vi "IsTimeToLaunchGSW__slk_mt.vi"(8 "error in (no error)":errorcluster) -> (0 "error out":errorcluster, 3 "ready?":bool)   [LabVIEW 2020]
doc: "Checks if it is ready to launch GSW."
panel:
  # "IsTimeToLaunchGSW__slk_mt.vi\nChecks if it is ready to launch GSW.\n\nNOTICE -- YOU MUST LEAVE THIS NOTICE IN PLACE.\n\nCopyright (c) 2011, LIANG LIU Shawn.Liu.cn@gmail.com\nAll rights reserved.\n\nRedistribution and use in source and binary forms, with or without modification, are permitted provided that the following conditions are met:\n-Redistributions of source code must retain the above copyright notice, this list of conditions and the following disclaimer.\n-Redistributions in binary form must reproduce the above copyright notice, this list of conditions and the following disclaimer in the documentation and/or other materials provided with the distribution.\n-Neither the name of the eLp nor the names of its contributors may be used to endorse or promote products derived from this software without specific prior written permission.\n\nTHIS SOFTWARE IS PROVIDED BY THE COPYRIGHT HOLDERS AND CONTRIBUTORS \"AS IS\" AND ANY EXPRESS OR IMPLIED WARRANTIES, INCLUDING, BUT NOT LIMITED TO, THE IMPLIED WARRANTIES OF MERCHANTABILITY AND FITNESS FOR A PARTICULAR PURPOSE ARE DISCLAIMED. IN NO EVENT SHALL THE COPYRIGHT HOLDER OR CONTRIBUTORS BE LIABLE FOR ANY DIRECT, INDIRECT, INCIDENTAL, SPECIAL, EXEMPLARY, OR CONSEQUENTIAL DAMAGES (INCLUDING, BUT NOT LIMITED TO, PROCUREMENT OF SUBSTITUTE GOODS OR SERVICES; LOSS OF USE, DATA, OR PROFITS; OR BUSINESS INTERRUPTION) HOWEVER CAUSED AND ON ANY THEORY OF LIABILITY, WHETHER IN CONTRACT, STRICT LIABILITY, OR TORT (INCLUDING NEGLIGENCE OR OTHERWISE) ARISING IN ANY WAY OUT OF THE USE OF THIS SOFTWARE, EVEN IF ADVISED OF THE POSSIBILITY OF SUCH DAMAGE."
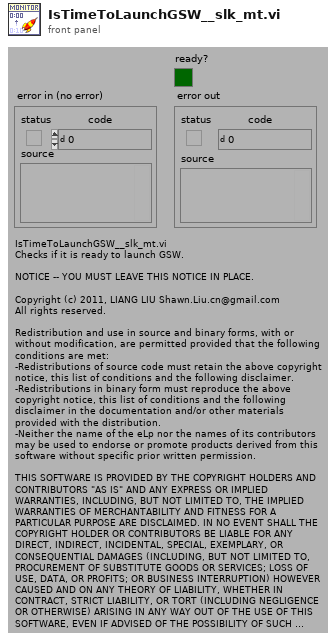
[diagram p1: front panel]
types:
  T1 = enum32{"Invalid", "Standard", "Closed", "Hidden", "Minimized", "Maximized"}
  T2 = typedef "VIMemory VI info.ctl" = cluster{"Project":string, "ComputingNode":string, "VI Name":string, "App Refnum":refnum<vi>}
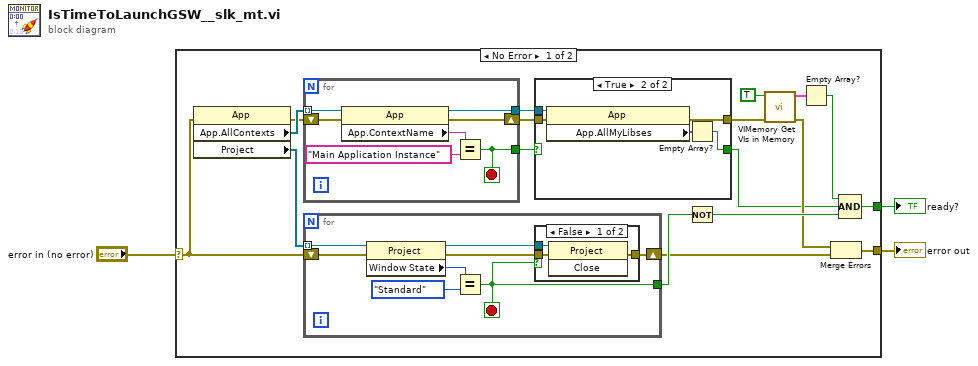
[diagram p0: block diagram]
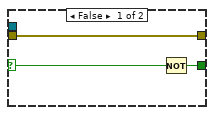
[diagram p3: hidden frame]
diagram:
  n1 = case shown="No Error" "error in (no error)" {
    selector: "error in (no error)" -> [w6 w49]
    tunnel: [w21 _] -> w3
    tunnel: [w5 w49] -> w1
    frame No Error {
      n2 = property class="App"(error in=w6) -> (error out=w19:errorcluster, "App.AllContexts"=w20:refnum<vi>[], "Project"=w14:refnum<vi>[])  [unwired: 1 in, 1 out]
      n3 = for {
        tunnel: w20 -> [w48] mode=indexing
        shift-right: [w46] -> w17
        shift-left: w19 -> [w47]
        tunnel: [w43] -> w16
        tunnel: [w42] -> w18
        stop <- w42 stop-if-true
        n4 = property class="App"(reference=w48, error in=w47) -> (reference out=w43:refnum<vi>, error out=w46:errorcluster, "App.ContextName"=w45:string)
        n5 = Equal?(x=w45, y="Main Application Instance") -> (x = y?=w42:bool)
      }
      n6 = for {
        tunnel: w14 -> [w29] mode=indexing
        shift-right: [w24] -> w4
        shift-left: w6 -> [w28]
        tunnel: [w23] -> w13
        stop <- w23 stop-if-true
        n7 = property class="Project"(reference=w29, error in=w28) -> (reference out=w22:refnum<vi>, error out=w25:errorcluster, "Window State"=w27:T1)
        n8 = Equal?(x=w27, y=T1."Standard") -> (x = y?=w23:bool)
        n9 = case shown="False" w23 {
          tunnel: w25 -> [w32 w33]
          tunnel: [w31 w33] -> w24
          tunnel: w22 -> [w30 _]
          frame False {
            n10 = invoke class="Project" method="Close"(reference=w30, error in=w32) -> (error out=w31:errorcluster)  [unwired: 1 in, 2 out]
          }
          frame True {
          }
        }
      }
      n11 = case "Ignore if do not find Main Application Instance context" shown="True" w18 {
        selector: w18 -> [w36 _]
        tunnel: w17 -> [w35 w40]
        tunnel: w16 -> [_ w41]
        tunnel: [w35 w38] -> w11
        tunnel: [w34 w37] -> w8
        frame False {
          n12 = Not(x=w36) -> (.not. x?=w34:bool)
        }
        frame True {
          n13 = property class="App"(reference=w41, error in=w40) -> (error out=w38:errorcluster, "App.AllMyLibses"=w39:string[])  [unwired: 1 out]
          n14 = Empty Array?(array=w39) -> (empty?=w37:bool)
        }
      }
      n15 = Not(x=w13) -> (.not. x?=w15:bool)
      n16 = call <vilib>:"VIMemory Get VIs in Memory.vi"("error in"=w11, "Only VIs with Open FPs?"=TRUE) -> ("error out"=w10:errorcluster, "VIs in memory"=w9:T2[])  [unwired: 8 in]
      n17 = Empty Array?(array=w9) -> (empty?=w7:bool)
      n18 = Merge Errors(w10, w4) -> (w5:errorcluster)
      n19 = Compound Arithmetic op=AND(w7, w8, w15) -> (w21:bool)
    }
    frame Error {
    }
  }
  "ready?" <- w3
  "error out" <- w1
